vi "CTRE_Logger_Open.vi"   [LabVIEW 2016]
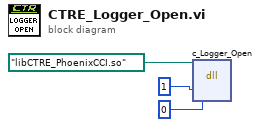
[diagram p0: block diagram]
diagram:
  n1 = dll-call lib="?" fn="c_Logger_Open"(path in=path "libCTRE_PhoenixCCI.so", "language"=1, "logDriverStation"=u8 0) -> ()  [unwired: 5 in, 2 out]
